vi "API - Config Button - No Error.vi"(8 "Error In":errorcluster, 11 "Error Button":refnum<vi>) -> (0 "Error Out":errorcluster)   [LabVIEW 2016, in "Error Manager.lvlib"]
doc: "Configures a button to indicate that no error has occurred, or that all errors have been marked as read\n1. Sets the background colour of the button to pale green RGB : 204, 255, 223\n2. Sets the 'Blinking' property to FALSE.\n3. Sets the Boolean Text of the button to 'No error'\n\nRecommended use: Poll the 'Have all errors been read' flag by calling 'Have all errors been read.vi' repeatedly. Call this VI when the flag is TRUE (no errors).\n\nNB. You can choose to never call this VI if you need to configure the button differently (different style, appearance) or if your app uses another method to reassure the user that all errors have been dealt with.\n\nError in behaviour: This VI skips execution (does not execute) if 'error in' contains an error."
uses:
  Error Manager.lvlib
  <vilib>/Utility/miscctls.llb/LVFontTypeDef.ctl
panel:
  # "Input\nInputs to the VI"
  # "Development\nControls or indicators that are useful for development or testing, but which are not outputs of the VI."
  # "Output\nOutputs of the VI"
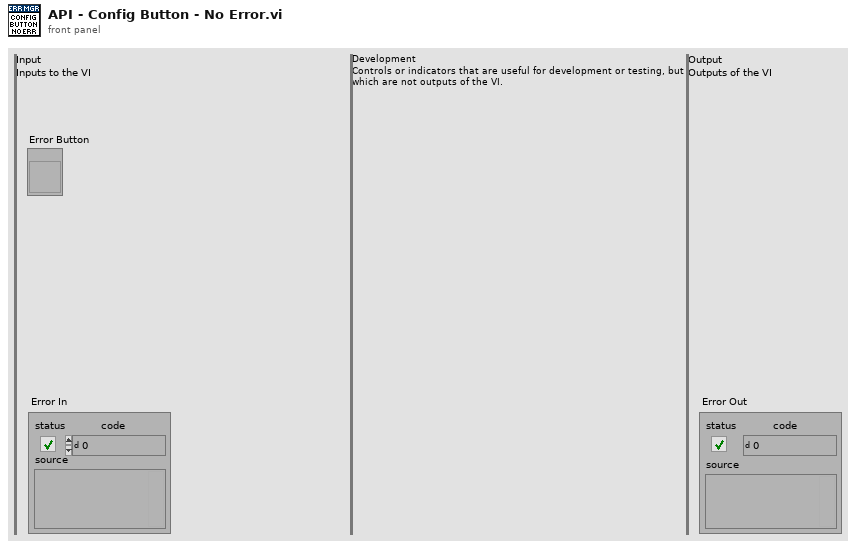
[diagram p1: front panel]
types:
  T1 = typedef "LVFontTypeDef.ctl" = cluster{"Font Name":string, "Size":u16, "Bold":bool, "Italic":bool, "Underline":bool, "Strikeout":bool, "Color":u32}
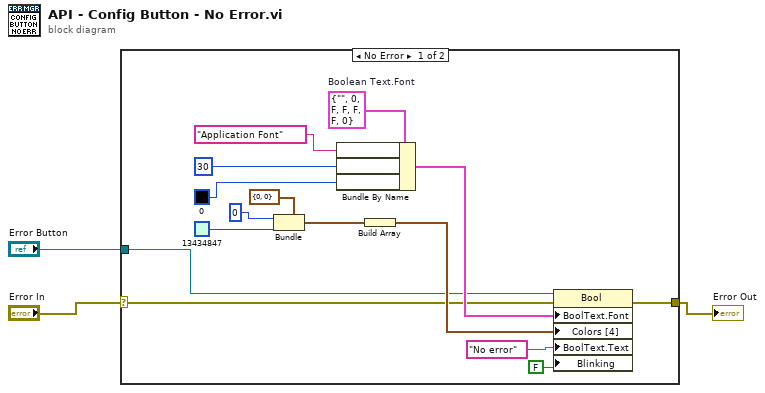
[diagram p0: block diagram]
diagram:
  n1 = case shown="No Error" "Error In" {
    selector: "Error In" -> [w6 w19]
    tunnel: [w5 w19] -> w2
    tunnel: "Error Button" -> [w4 _]
    frame No Error {
      w12 = T1 {"Font Name"="", "Size"=0, "Bold"=FALSE, "Italic"=FALSE, "Underline"=FALSE, "Strikeout"=FALSE, "Color"=0}  # Boolean Text.Font
      n2 = Bundle(cluster=cluster{u32, u32} {0, 0}, u32 0, u32 13434847) -> (w17:cluster{u32, u32})
      n3 = Bundle By Name(cluster=w12, "Application Font" ("Font Name"), u16 30 ("Size"), u32 0) -> (w16:T1)
      n4 = Build Array(w17) -> (w18:cluster{u32, u32}[])
      n5 = property on="Property Node" class="Bool"(reference=w4, error in=w6, "BoolText.Font"=w16, "Colors [4]"=w18, "BoolText.Text"="No error" ("Boolean Text.Text"), "Blinking"=FALSE) -> (error out=w5:errorcluster)  [unwired: 1 out]
    }
    frame Error {
    }
  }
  "Error Out" <- w2
